vi "AviTrack2pointsTreshold.vi"() -> ()   [LabVIEW 2015]
uses:
  <vilib>/vision/Image Controls.llb/IMAQ Image.ctl
  <vilib>/vision/NI_Vision_Development_Module.lvlib
panel:
  out "error out":errorcluster
  out "Progress Bar 2":i32(slide) max=25 scale=-1.0..205.0
  in  "base path 2":path
  in  "Color Mode":u16(ring) items=["RGB", "HSL", "HSV", "HSI"]
  in  "Red or Hue Range":cluster{"Lower value":i32, "Upper value":i32}={"Lower value"=0, "Upper value"=255}
  in  "Green or Sat Range":cluster{"Lower value":i32, "Upper value":i32}={"Lower value"=0, "Upper value"=255}
  in  "Blue or Luma or Val or Inten Range":cluster{"Lower value":i32, "Upper value":i32}={"Lower value"=0, "Upper value"=255}
  out "Image":T1(plugin-control)
  in  "stop":bool
  out "Image Dst Out":T1
  out "Image 2":T1(plugin-control)
  in  "invert":bool
  out "ITemplate":T1(plugin-control)
  out "error out 2":errorcluster
  out "ITemplate 2":T1(plugin-control)
  in  "GetTemplate":bool
  out "IMA 2":T1(plugin-control)
  in  "Color":u32(colorbox)=16711680
  in  "Color 2":u32(colorbox)=16711680
  in  "Font, Size & Style":T2={"Desired Font (Application)"=enum."Application Font", "[User-specified Font]"={"Font Name"="", "Size"=12, "Strikeout?"=FALSE, "Italic?"=FALSE, "Underline?"=FALSE, "Outline?"=FALSE, "Shadow?"=FALSE, "Bold?"=FALSE, "Rotation Angle"=0.0}, "Horizontal Alignment"=0, "Vertical Alignment"=0} {"Vertical Alignment" items=["Bottom", "Top", "Baseline"]; "Horizontal Alignment" items=["Left", "Center", "Right"]; "[User-specified Font]"."Rotation Angle" format="%.2f"}
  in  "Origin":cluster{"X":i32, "Y":i32}
  in  "SetTemplate 2":bool
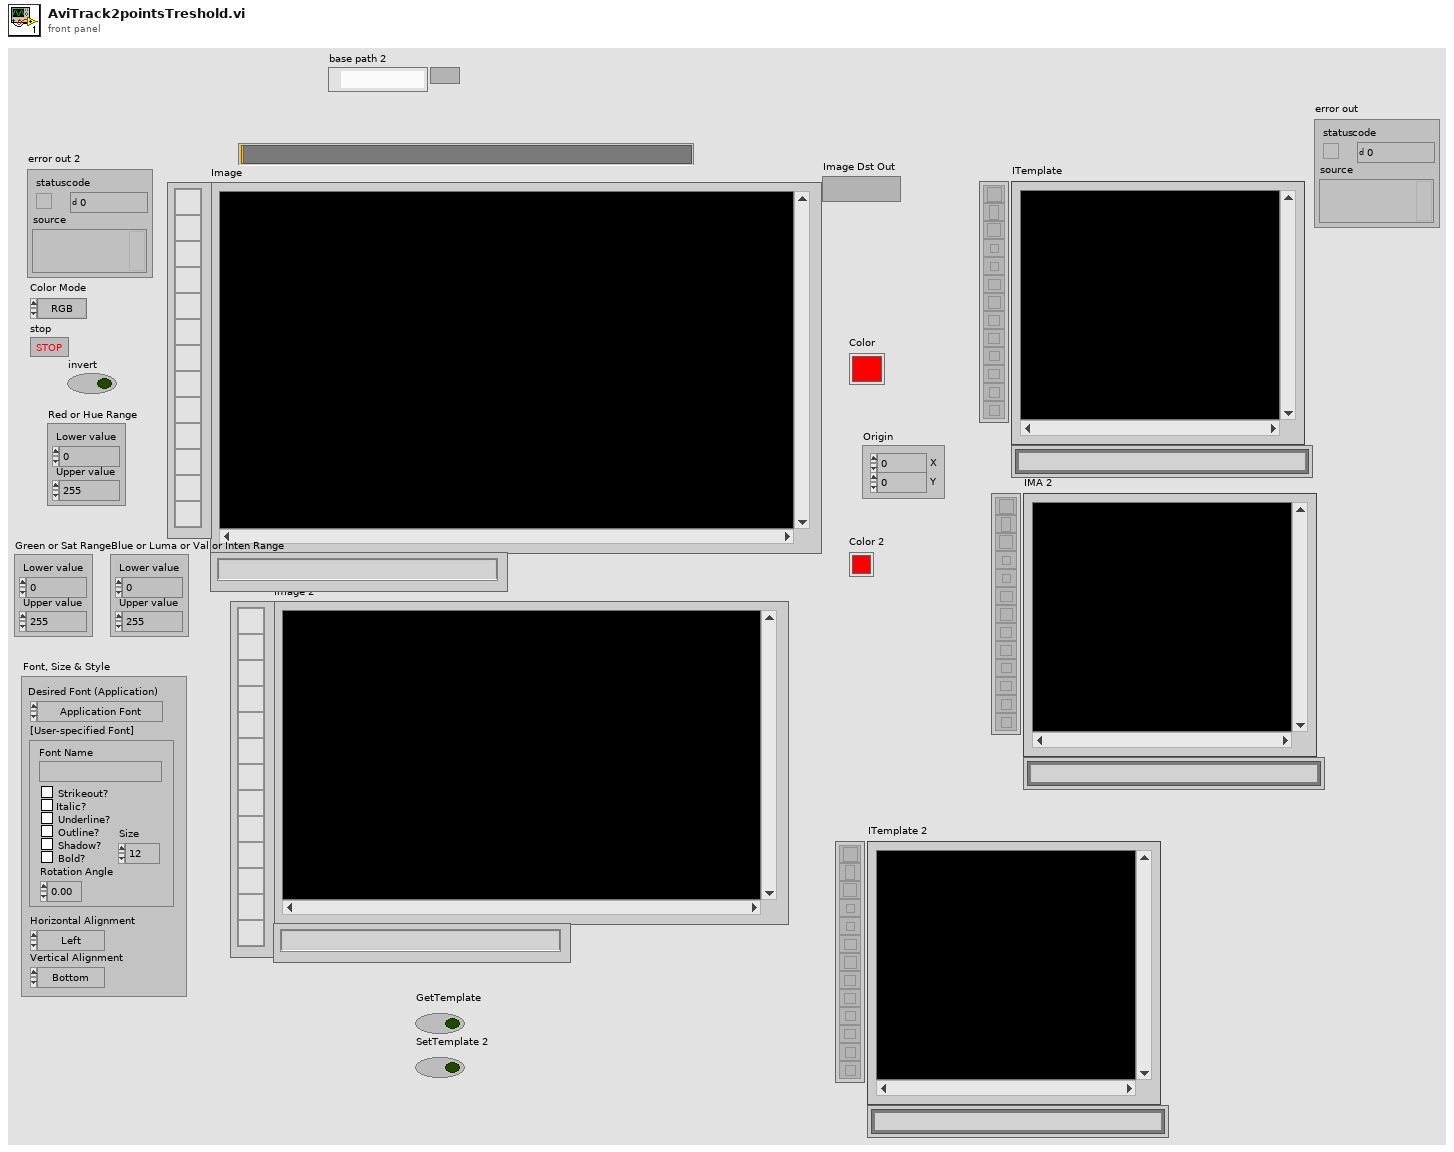
[diagram p1: front panel]
types:
  T1 = typedef "IMAQ Image.ctl" = refnum<image>
  T2 = cluster{"Desired Font (Application)":enum16{"User-specified Font", "Application Font", "System Font", "Dialog Font"}, "[User-specified Font]":cluster{"Font Name":string, "Size":i16, "Strikeout?":bool, "Italic?":bool, "Underline?":bool, "Outline?":bool, "Shadow?":bool, "Bold?":bool, "Rotation Angle":dbl}, "Horizontal Alignment":i16, "Vertical Alignment":i16}
  T3 = typedef "Image Type" = u32
  T4 = typedef "IMAQ AVI2 Refnum.ctl" = refnum<k20>
  T5 = cluster{"Width":u32, "Height":u32, "Frames Per Second":u32, "Codec":string, "Has Data":bool}
  T6 = cluster{"Global Rectangle":i32[], "Contours":cluster{"Contour Type":u32, "ROI Type":u32, "Points":i32[]}[]}
  T7 = typedef "IMAQ Rectangle" = cluster{"Left":i32, "Top":i32, "Right":i32, "Bottom":i32, "Rotation":dbl}
  T8 = cluster{"Position":cluster{"x":sgl, "y":sgl}, "Angle":sgl, "Scale":sgl, "Score":sgl, "Bounding Box":cluster{"x":sgl, "y":sgl}[]}[]
  T9 = cluster{"Matches[0]":cluster{"Position":cluster{"x":sgl, "y":sgl}, "Angle":sgl, "Scale":sgl, "Score":sgl, "Bounding Box":cluster{"x":sgl, "y":sgl}[]}, "Matches[1]":cluster{"Position":cluster{"x":sgl, "y":sgl}, "Angle":sgl, "Scale":sgl, "Score":sgl, "Bounding Box":cluster{"x":sgl, "y":sgl}[]}, "Matches[2]":cluster{"Position":cluster{"x":sgl, "y":sgl}, "Angle":sgl, "Scale":sgl, "Score":sgl, "Bounding Box":cluster{"x":sgl, "y":sgl}[]}, "Matches[3]":cluster{"Position":cluster{"x":sgl, "y":sgl}, "Angle":sgl, "Scale":sgl, "Score":sgl, "Bounding Box":cluster{"x":sgl, "y":sgl}[]}, "Matches[4]":cluster{"Position":cluster{"x":sgl, "y":sgl}, "Angle":sgl, "Scale":sgl, "Score":sgl, "Bounding Box":cluster{"x":sgl, "y":sgl}[]}, "Matches[5]":cluster{"Position":cluster{"x":sgl, "y":sgl}, "Angle":sgl, "Scale":sgl, "Score":sgl, "Bounding Box":cluster{"x":sgl, "y":sgl}[]}, "Matches[6]":cluster{"Position":cluster{"x":sgl, "y":sgl}, "Angle":sgl, "Scale":sgl, "Score":sgl, "Bounding Box":cluster{"x":sgl, "y":sgl}[]}, "Matches[7]":cluster{"Position":cluster{"x":sgl, "y":sgl}, "Angle":sgl, "Scale":sgl, "Score":sgl, "Bounding Box":cluster{"x":sgl, "y":sgl}[]}, "Matches[8]":cluster{"Position":cluster{"x":sgl, "y":sgl}, "Angle":sgl, "Scale":sgl, "Score":sgl, "Bounding Box":cluster{"x":sgl, "y":sgl}[]}}
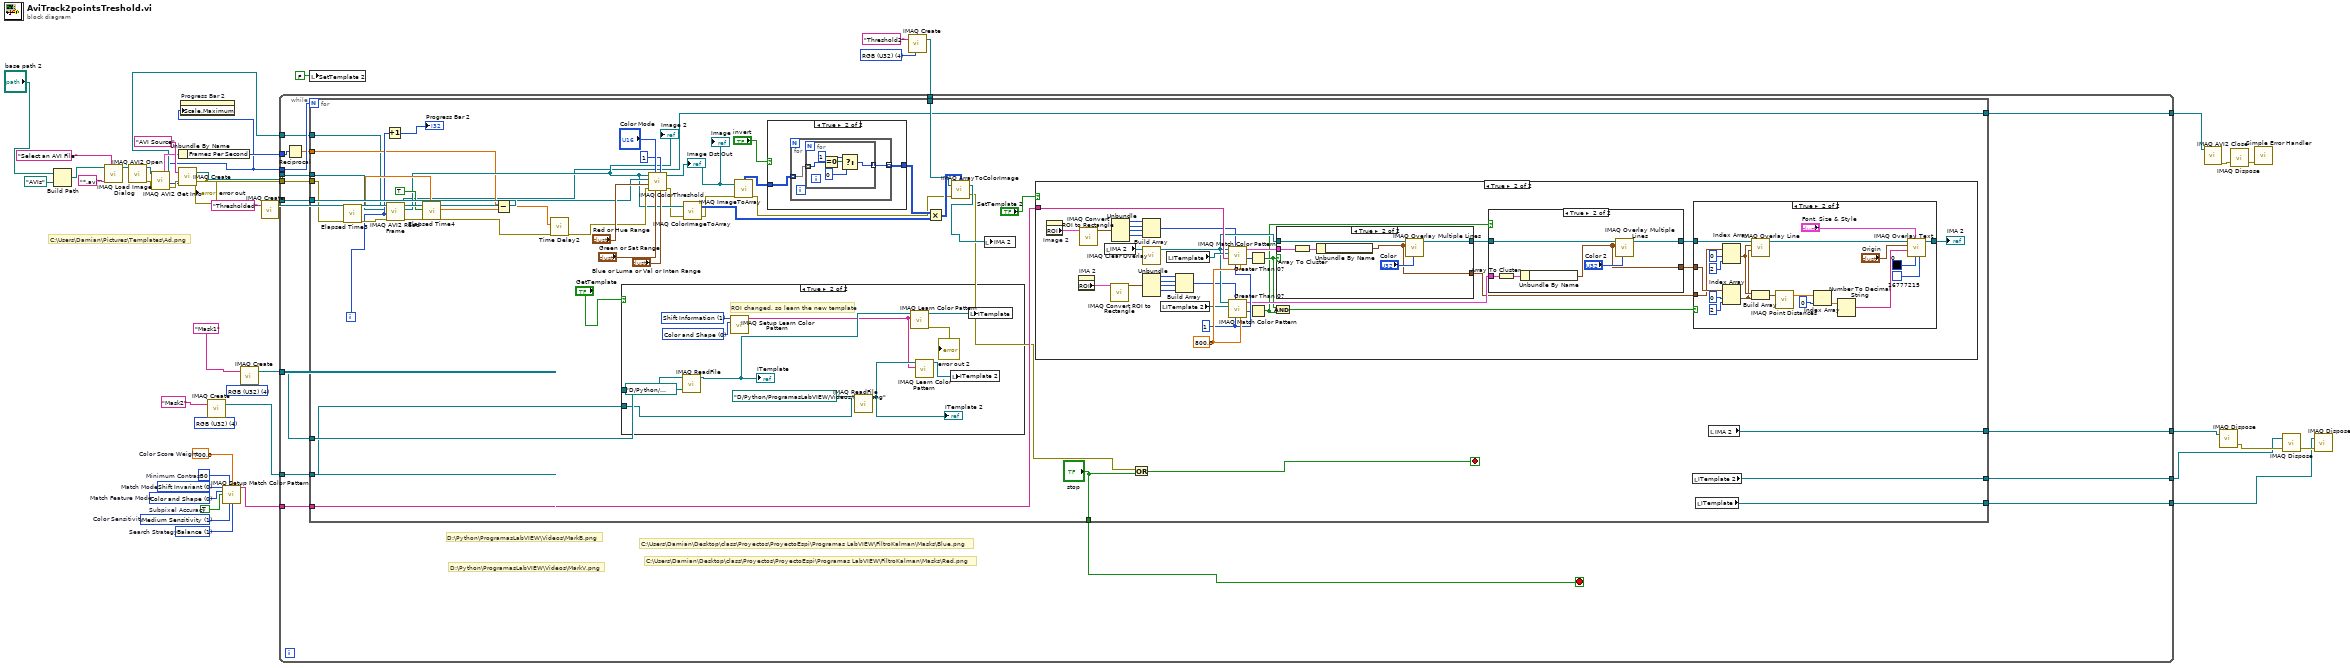
[diagram p0: block diagram]
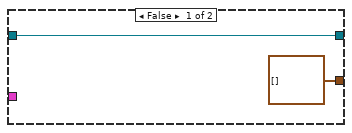
[diagram p4: hidden frame]
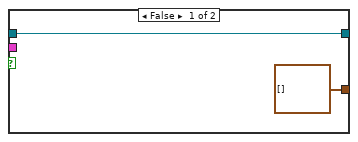
[diagram p5: hidden frame]
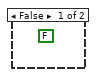
[diagram p6: hidden frame]
diagram:
  w6 = T3 4 items=["Grayscale (U8)", "Grayscale (I16)", "Grayscale (SGL)", "Complex (CSG)", "RGB (U32)", "HSL (U32)", "RGB (U64)", "Grayscale (U16)"] ("Image Type")
  w35 = T3 4 items=["Grayscale (U8)", "Grayscale (I16)", "Grayscale (SGL)", "Complex (CSG)", "RGB (U32)", "HSL (U32)", "RGB (U64)", "Grayscale (U16)"] ("Image Type")
  w37 = T3 4 items=["Grayscale (U8)", "Grayscale (I16)", "Grayscale (SGL)", "Complex (CSG)", "RGB (U32)", "HSL (U32)", "RGB (U64)", "Grayscale (U16)"] ("Image Type")
  w43 = TRUE  # Subpixel Accuracy
  w45 = u32 0 items=["Color and Shape", "Color", "Shape"]  # Match Feature Mode
  w39 = u32 1 items=["Conservative", "Balance", "Aggressive", "Very Aggressive"]  # Search Strategy
  w41 = 50  # Minimum Contrast
  w42 = sgl 700.0  # Color Score Weight
  w40 = u32 1 items=["Low Sensitivity", "Medium Sensitivity", "High Sensitivity"]  # Color Sensitivity
  w44 = u32 0 items=["Shift Invariant", "Rotation Invariant"]  # Match Mode
  # "C:\\Users\\Damian\\Pictures\\Templates\\Ad.png"
  n1 = Build Path(base path="base path 2", name or relative path=path "AVIs") -> (appended path=w14:path)
  n2 = call "IMAQ Load Image Dialog"("Prompt"="Select an AVI File" ("prompt"), "Pattern"="*.avi", "Start Path"=w14) -> ("Path"=w13:path)  [unwired: 6 in, 2 out]
  n3 = call "IMAQ AVI2 Open"("AVI File Path"=w13) -> ("error out"=w20:errorcluster, "AVI Refnum"=w19:T4)  [unwired: 2 in, 7 out]
  n4 = call "IMAQ AVI2 Get Info"("error in (no error)"=w20, "AVI Refnum"=w19) -> ("error out"=w18:errorcluster, "Image Type"=w17:T3, "Number of Frames"=w2:u32, "AVI Refnum (duplicate)"=w8:T4, "Frame Data"=w21:T5)  [unwired: 5 out]
  n5 = Unbundle By Name(w21) -> ("Frames Per Second"=w7:u32)
  n6 = call "IMAQ Create"("Image Name"="AVI Source", "Image Type"=w17, "error in (no error)"=w18) -> ("New Image"=w10:T1, "error out"=w9:errorcluster)  [unwired: 1 in, 1 out]
  "error out" <- w9
  n7 = property on="Progress Bar 2" class="Slide (strict)"("Scale.Maximum"=w2) -> ()  [unwired: 2 in, 2 out]
  n8 = call "IMAQ Create"("Image Name"="Mask2", "Image Type"=w35) -> ("New Image"=w31:T1)  [unwired: 3 in, 1 out]
  n9 = call "IMAQ Setup Match Color Pattern"("Match Mode"=w44, "Minimum Contrast"=w41, "Color Score Weight"=w42, "Match Feature Mode"=w45, "Subpixel Accuracy"=w43, "Color Sensitivity"=w40, "Search Strategy"=w39) -> ("Match Color Pattern Setup Data"=w30:string)  [unwired: 7 in, 1 out]
  n10 = call "IMAQ Create"("Image Name"="Mask1", "Image Type"=w37) -> ("New Image"=w32:T1)  [unwired: 3 in, 1 out]
  n11 = call "IMAQ Create"("Image Name"="Thresholded") -> ("New Image"=w33:T1)  [unwired: 3 in, 2 out]
  n12 = local write "SetTemplate 2"(FALSE ("SetTemplate 2")) -> ()
  n13 = call "IMAQ Create"("Image Name"="Threshold2", "Image Type"=w6) -> ("New Image"=w4:T1)  [unwired: 2 in, 2 out]
  n14 = while {
    tunnel: w32 -> [w61]
    tunnel: w31 -> [w60]
    tunnel: w30 -> [w59]
    tunnel: w33 -> [w58]
    tunnel: [w57] -> w27
    tunnel: [w56] -> w26
    tunnel: [w55] -> w25
    tunnel: w10 -> [w54]
    tunnel: w9 -> [w53]
    tunnel: w8 -> [w46]
    tunnel: w2 -> [w52]
    tunnel: w7 -> [w51]
    tunnel: w4 -> [w48]
    tunnel: [w47] -> w3
    stop <- w49 stop-if-true
    # "D:\\Python\\ProgramasLabVIEW\\Videos\\MarkV.png"
    # "D:\\Python\\ProgramasLabVIEW\\Videos\\MarkB.png"
    # "C:\\Users\\Damian\\Desktop\\class\\Proyectos\\ProyectoEspi\\Programas LabVIEW\\FiltroKalman\\Masks\\Red.png"
    # "C:\\Users\\Damian\\Desktop\\class\\Proyectos\\ProyectoEspi\\Programas LabVIEW\\FiltroKalman\\Masks\\Blue.png"
    n15 = Reciprocal(x=w51) -> (1/x=w50:dbl)
    n16 = for {
      N: w52 -> [_]
      tunnel: w61 -> [w94]
      tunnel: w60 -> [w93]
      tunnel: w59 -> [w91]
      tunnel: w58 -> [w90]
      tunnel: [w89] -> w57
      tunnel: [w88] -> w56
      tunnel: [w87] -> w55
      tunnel: w54 -> [w62]
      tunnel: w53 -> [w77]
      tunnel: w50 -> [w72]
      tunnel: ["stop"] -> w49
      tunnel: w48 -> [w67]
      tunnel: [w64] -> w47
      tunnel: w46 -> [w63]
      i -> [w75]
      stop <- w68 stop-if-true
      n17 = call "Elapsed Time3"("error in (no error)"=w77) -> ("Present (s)"=w83:dbl, "error out"=w84:errorcluster)  [unwired: 11 in, 6 out]
      n18 = Increment(x=w75) -> (x+1=→"Progress Bar 2":i32)
      n19 = call "IMAQ AVI2 Read Frame"("error in (no error)"=w84, "Frame Number"=w75, "Image"=w62, "AVI Refnum"=w63) -> ("error out"=w81:errorcluster, "Image Out"=w74:T1, "AVI Refnum (duplicate)"=w64:T4)  [unwired: 5 out]
      "Image 2" <- w74
      n20 = call "Elapsed Time4"("Reset"=TRUE, "error in (no error)"=w81, "Set Start Time (s)"=w83) -> ("Elapsed Time (s)"=w80:dbl, "error out"=w79:errorcluster)  [unwired: 9 in, 6 out]
      n21 = Subtract(x=w72, y=w80) -> (x-y=w73:dbl)
      n22 = call "Time Delay2"("error in (no error)"=w79, "Delay Time (s)"=w73) -> ("error out"=w76:errorcluster)  [unwired: 9 in]
      n23 = case shown="True" "GetTemplate" {
        tunnel: w94 -> [_ w181]
        tunnel: w93 -> [_ w177]
        frame False {
          (unwired) FALSE ("SetTemplate 2")
        }
        frame True {
          w186 = u32 0 items=["Color and Shape", "Color", "Shape "] ("Feature Mode")
          w187 = u32 1 items=["All", "Shift Information", "Rotation Information"] ("Learn Mode")
          # "ROI changed, so learn the new template"
          n24 = call "IMAQ ReadFile"("File Path"=path "D:/Python/ProgramasLabVIEW/Videos/Gris.png", "Image"=w181) -> ("Image Out"=w182:T1)  [unwired: 5 in, 4 out]
          "ITemplate" <- w182
          n25 = call "IMAQ Setup Learn Color Pattern"("Feature Mode"=w186, "Learn Mode"=w187) -> ("Learn Color Pattern Setup Data"=w178:string)  [unwired: 8 in, 1 out]
          n26 = call "IMAQ ReadFile"("File Path"=path "D:/Python/ProgramasLabVIEW/Videos/Black.png", "Image"=w177) -> ("Image Out"=w179:T1)  [unwired: 5 in, 4 out]
          "ITemplate 2" <- w179
          n27 = call "IMAQ Learn Color Pattern"("Learn Color Pattern Setup Data"=w178, "Image"=w182) -> ("error out"=→"error out 2":errorcluster, "Template Image Out"=w184:T1)  [unwired: 8 in]
          n28 = call "IMAQ Learn Color Pattern"("Learn Color Pattern Setup Data"=w178, "Image"=w179) -> ("Template Image Out"=w176:T1)  [unwired: 8 in, 1 out]
          n29 = local write "ITemplate 2"(w176) -> ()
          n30 = local write "ITemplate"(w184) -> ()
        }
      }
      n31 = call "IMAQ ColorThreshold"("Blue or Luma or Val or Inten Range"="Blue or Luma or Val or Inten Range", "Replace Value"=1, "Green or Sat Range"="Green or Sat Range", "Color Mode"="Color Mode", "error in (no error)"=w76, "Red or Hue Range"="Red or Hue Range", "Image Dst"=w90, "Image Src"=w74) -> ("error out"=w71:errorcluster, "Image Dst Out"=w100:T1)  [unwired: 2 in]
      "Image" <- w100
      "Image Dst Out" <- w100
      n32 = call "IMAQ ColorImageToArray"("Image"=w74, "error in (no error)"=w71) -> ("Image Pixels (U32)"=w97:u32[][], "error out"=w70:errorcluster)  [unwired: 2 in, 1 out]
      n33 = call "IMAQ ImageToArray"("error in (no error)"=w70, "Image"=w100) -> ("error out"=w66:errorcluster, "Image Pixels (U8)"=w95:u8[][])  [unwired: 2 in, 3 out]
      n34 = case shown="True" "invert" {
        tunnel: w95 -> [w188 w190]
        tunnel: [w188 w189] -> w98
        frame False {
        }
        frame True {
          n35 = for {
            tunnel: w190 -> [w192] mode=indexing
            tunnel: [w191] -> w189 mode=indexing
            n36 = for {
              tunnel: w192 -> [w193] mode=indexing
              tunnel: [w194] -> w191 mode=indexing
              n37 = Equal To 0?(x=w193) -> (x = 0?=w197:bool)
              n38 = Select(t=1, s=w197, f=0) -> (s? t:f=w194:i32)
            }
          }
        }
      }
      n39 = Multiply(x=w98, y=w97) -> (x*y=w96:u32[][])
      n40 = call "IMAQ ArrayToColorImage"("Image Pixels (U32)"=w96, "Image"=w67, "error in (no error)"=w66) -> ("Image Out"=w85:T1, "error out"=w65:errorcluster)  [unwired: 2 in]
      n41 = local write "IMA 2"(w85) -> ()
      n42 = case shown="True" "SetTemplate 2" {
        tunnel: w91 -> [_ w138]
        frame False {
        }
        frame True {
          w132 = 1 ("Number of Matches Requested")
          w133 = sgl 800.0 ("Minimum Match Score")
          n43 = property on="Image 2" class="ImageControl"() -> ("ROI"=w107:T6)  [unwired: 2 in, 2 out]
          n44 = property on="IMA 2" class="ImageControl"() -> ("ROI"=w106:T6)  [unwired: 2 in, 2 out]
          n45 = call "IMAQ Convert ROI to Rectangle"("ROI Descriptor"=w107) -> ("Rectangle"=w119:T7)  [unwired: 8 in, 1 out]
          n46 = local read "IMA 2"() -> (w136:T1)
          n47 = call "IMAQ Convert ROI to Rectangle"("ROI Descriptor"=w106) -> ("Rectangle"=w113:T7)  [unwired: 8 in, 1 out]
          n48 = Unbundle(w119) -> ("Left"=w118:i32, "Top"=w117:i32, "Right"=w115:i32, "Bottom"=w114:i32)  [unwired: 1 out]
          n49 = Build Array(w118, w117, w115, w114) -> (w116:i32[])
          n50 = call "IMAQ Clear Overlay"("Image"=w136) -> ("Image Out"=w130:T1)  [unwired: 9 in, 1 out]
          n51 = Unbundle(w113) -> ("Left"=w112:i32, "Top"=w111:i32, "Right"=w110:i32, "Bottom"=w109:i32)  [unwired: 1 out]
          n52 = local read "ITemplate 2"() -> (w131:T1)
          n53 = local read "ITemplate"() -> (w137:T1)
          n54 = Build Array(w112, w111, w110, w109) -> (w108:i32[])
          n55 = call "IMAQ Match Color Pattern"("Minimum Match Score"=w133, "Number of Matches Requested"=w132, "Optional Rectangle"=w116, "Match Color Pattern Setup Data"=w138, "Template Image"=w137, "Image"=w130) -> ("Number of Matches"=w134:i32, "Matches"=w135:T8)  [unwired: 3 in, 1 out]
          n56 = call "IMAQ Match Color Pattern"("Minimum Match Score"=w133, "Number of Matches Requested"=w132, "Optional Rectangle"=w108, "Template Image"=w131, "Image"=w130) -> ("Number of Matches"=w129:i32, "Matches"=w128:T8)  [unwired: 4 in, 1 out]
          n57 = Greater Than 0?(x=w134) -> (x > 0?=w126:bool)
          n58 = Greater Than 0?(x=w129) -> (x > 0?=w125:bool)
          n59 = And(x=w126, y=w125) -> (x .and. y?=w123:bool)
          n60 = case shown="True" w126 {
            tunnel: w135 -> [_ w175]
            tunnel: w130 -> [w169 w174]
            tunnel: [w169 w171] -> w127
            tunnel: [cluster{"x":sgl, "y":sgl}[] [] ("Bounding Box") w170] -> w124
            frame False {
            }
            frame True {
              n61 = Array To Cluster(array=w175) -> (cluster=w172:T9)
              n62 = Unbundle By Name(w172) -> ("Matches[0].Bounding Box"=w170:cluster{"x":sgl, "y":sgl}[])
              n63 = call "IMAQ Overlay Multiple Lines"("Color"="Color", "Line End Points"=w170, "Image"=w174) -> ("Image Out"=w171:T1)  [unwired: 3 in, 5 out]
            }
          }
          n64 = case shown="True" w125 {
            tunnel: w128 -> [_ w165]
            tunnel: w127 -> [w161 w164]
            tunnel: [w161 w163] -> w121
            tunnel: [cluster{"x":sgl, "y":sgl}[] [] ("Bounding Box") w162] -> w122
            frame False {
            }
            frame True {
              n65 = Array To Cluster(array=w165) -> (cluster=w167:T9)
              n66 = Unbundle By Name(w167) -> ("Matches[0].Bounding Box"=w162:cluster{"x":sgl, "y":sgl}[])
              n67 = call "IMAQ Overlay Multiple Lines"("Color"="Color 2", "Line End Points"=w162, "Image"=w164) -> ("Image Out"=w163:T1)  [unwired: 3 in, 5 out]
            }
          }
          n68 = case shown="True" w123 {
            tunnel: w124 -> [_ w156]
            tunnel: w122 -> [_ w158]
            tunnel: w121 -> [w139 w153]
            tunnel: [w139 w147] -> w120
            frame False {
            }
            frame True {
              n69 = Index Array(array=w156, index #1=0 ("index"), index #2=2 ("index")) -> (element #1=w152:cluster{"x":sgl, "y":sgl})  [unwired: 1 out]
              n70 = Index Array(array=w158, index #1=0 ("index"), index #2=2 ("index")) -> (element #1=w151:cluster{"x":sgl, "y":sgl})  [unwired: 1 out]
              n71 = call "IMAQ Overlay Line"("End Point"=w151, "Start Point"=w152, "Image"=w153) -> ("Image Out"=w148:T1)  [unwired: 7 in, 1 out]
              n72 = Build Array(w152, w151) -> (w150:cluster{"x":sgl, "y":sgl}[])
              n73 = call "IMAQ Point Distances"("Points"=w150) -> ("Distances"=w143:sgl[])  [unwired: 4 in, 1 out]
              n74 = Index Array(array=w143, index=0) -> (element=w141:sgl)
              n75 = Number To Decimal String(number=w141) -> (decimal integer string=w149:string)  [unwired: 1 in]
              n76 = call "IMAQ Overlay Text"("BG Color (Transparent)"=u32 16777215, "Text Color (black)"=u32 0, "Font, Size & Style"="Font, Size & Style", "String"=w149, "Origin"="Origin", "Image"=w148) -> ("Image Out"=w147:T1)  [unwired: 4 in, 1 out]
            }
          }
          "IMA 2" <- w120
        }
      }
      n77 = Or(x=w65, y="stop") -> (x .or. y?=w68:bool)
      n78 = local read "ITemplate 2"() -> (w88:T1)
      n79 = local read "ITemplate"() -> (w87:T1)
      n80 = local read "IMA 2"() -> (w89:T1)
    }
  }
  n81 = call "IMAQ AVI2 Close"("AVI Refnum"=w3) -> ("error out"=w23:errorcluster)  [unwired: 1 in, 9 out]
  n82 = call "IMAQ Dispose"("Image"=w27) -> ("error out"=w28:errorcluster)  [unwired: 5 in]
  n83 = call "IMAQ Dispose"("error in (no error)"=w23) -> ("error out"=w24:errorcluster)  [unwired: 2 in, 3 out]
  n84 = call <vilib>:"Simple Error Handler.vi"("error in (no error)"=w24) -> ()  [unwired: 1 in, 8 out]
  n85 = call "IMAQ Dispose"("Image"=w26, "error in (no error)"=w28) -> ("error out"=w29:errorcluster)  [unwired: 4 in]
  n86 = call "IMAQ Dispose"("Image"=w25, "error in (no error)"=w29) -> ()  [unwired: 4 in, 1 out]
